vi "Get Ball Angle.vi"(2 "Camera Res Y":i32, 3 "Camera Res X":i32, 4 "Ranked Objects":T1(array[cluster]) {"Score" format="%#.1g"}) -> (0 "Angle Y":dbl, 1 "Angle X":dbl)   [LabVIEW 2013]
doc: "Convert the center coordinates of the ball, on the interval [0, Camera Res X], [0, Camera Res Y] with (0, 0) being the top left to degrees with the center as the origin.\nUp and right are positive angles, down and left are negative."
panel:
  in  "Camera FOV Y":dbl=50.0
  in  "Camera FOV X":dbl=67.0
  # "Make sure these are accurate for the camera that is being used.\n67 x 50 for the M1103 (New camera)"
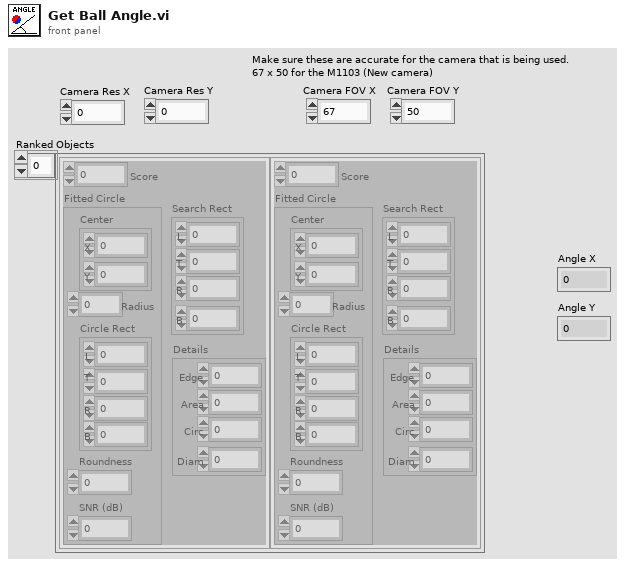
[diagram p1: front panel]
types:
  T1 = cluster{"Score":sgl, "Fitted Circle":cluster{"Center":cluster{"X":sgl, "Y":sgl}, "Radius":dbl, "Circle Rect":cluster{"L":sgl, "T":sgl, "R":sgl, "B":sgl}, "Roundness":dbl, "SNR (dB)":dbl}, "Search Rect":cluster{"L":sgl, "T":sgl, "R":sgl, "B":sgl}, "Details":cluster{"Edge":sgl, "Area":sgl, "Circ":sgl, "Diam":sgl}}[]
  T2 = cluster{"Score":sgl, "Fitted Circle":cluster{"Center":cluster{"X":sgl, "Y":sgl}, "Radius":dbl, "Circle Rect":cluster{"L":sgl, "T":sgl, "R":sgl, "B":sgl}, "Roundness":dbl, "SNR (dB)":dbl}, "Search Rect":cluster{"L":sgl, "T":sgl, "R":sgl, "B":sgl}, "Details":cluster{"Edge":sgl, "Area":sgl, "Circ":sgl, "Diam":sgl}}
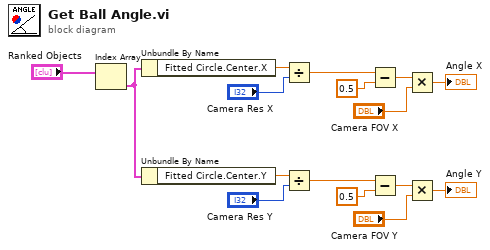
[diagram p0: block diagram]
diagram:
  n1 = Index Array(array="Ranked Objects") -> (element=w1:T2)  [unwired: 1 in]
  n2 = Unbundle By Name(w1) -> ("Fitted Circle.Center.X"=w11:sgl)
  n3 = Unbundle By Name(w1) -> ("Fitted Circle.Center.Y"=w4:sgl)
  n4 = Divide(x=w11, y="Camera Res X") -> (x/y=w15:sgl)
  n5 = Divide(x=w4, y="Camera Res Y") -> (x/y=w8:sgl)
  n6 = Subtract(x=w15, y=0.5) -> (x-y=w13:dbl)
  n7 = Subtract(x=w8, y=0.5) -> (x-y=w6:dbl)
  n8 = Multiply(x=w13, y="Camera FOV X") -> (x*y=→"Angle X":dbl)
  n9 = Multiply(x=w6, y="Camera FOV Y") -> (x*y=→"Angle Y":dbl)
